vi "1.1.vi"(8 "error in (no error)":errorcluster, 10 "input":string) -> (0 "error out":errorcluster, 2 "Out":dbl)   [LabVIEW 2017]
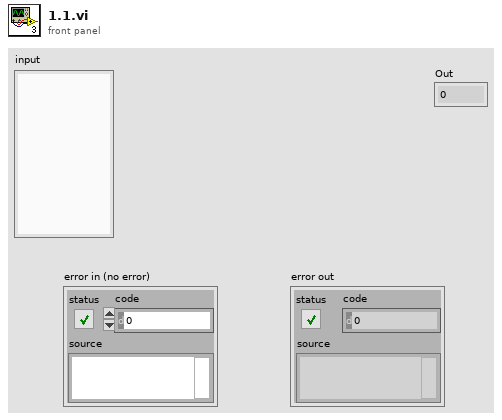
[diagram p1: front panel]
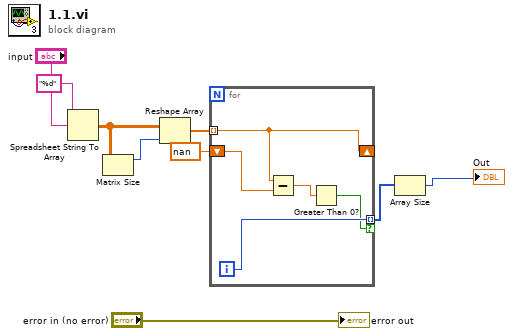
[diagram p0: block diagram]
diagram:
  n1 = Spreadsheet String To Array(format string="%d" ("delimiter (Tab)"), spreadsheet string="input") -> (array=w6:dbl[][])  [unwired: 2 in]
  n2 = Matrix Size(0:w6) -> (1:w5:i32)  [unwired: 1 out]
  n3 = Reshape Array(w6, w5) -> (w4:dbl[])
  n4 = for {
    tunnel: w4 -> [w14] mode=indexing
    shift-right: [w14] -> _
    shift-left: nan -> [w13]
    tunnel: [w11] -> w2 mode=indexing if=w10
    i -> [w11]
    n5 = Subtract(x=w14, y=w13) -> (x-y=w12:dbl)
    n6 = Greater Than 0?(x=w12) -> (x > 0?=w10:bool)
  }
  n7 = Array Size(array=w2) -> (size(s)=→"Out":i32)
  "error out" <- "error in (no error)"
